vi "Iterator.vi"(8 "error in":errorcluster, 11 "Iterator Actor in":refnum<class "Iterator NR Actor.lvclass">) -> (0 "error out":errorcluster, 3 "Iterator Actor out":refnum<class "Iterator NR Actor.lvclass">)   [LabVIEW 2023, in "Iterator Actor.lvlib" / "Iterator NR Actor.lvclass"]
doc: "(<B>Filename</B>: Actor Framework.lvlib:Actor.lvclass:Actor Core.vi)\n\nReceives messages to the actor, reacts to them, and initiates any error handling that may shut the actor down.\n\nDescendant classes may override this VI to append parallel tasks for the actor to complete while it handles messages. Overrides use the Call Parent Method node."
uses:
  Iterator NR Actor.lvclass
  Iterator NR Actor.lvclass/Iterator NR Actor.ctl
  Abstract Iterator Actor/Abstract Iterator Actor.lvclass
  <userlib>/_OpenG.lib/error/error.llb/openg_error.lvlib
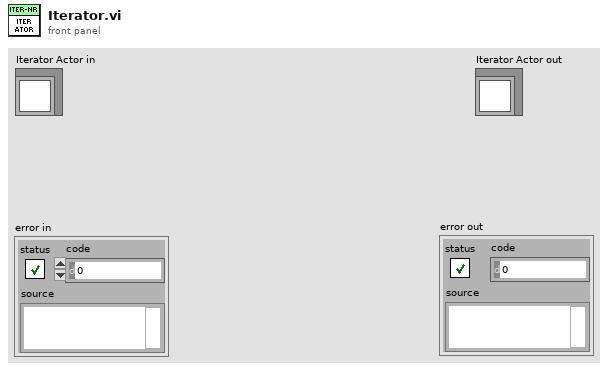
[diagram p1: front panel]
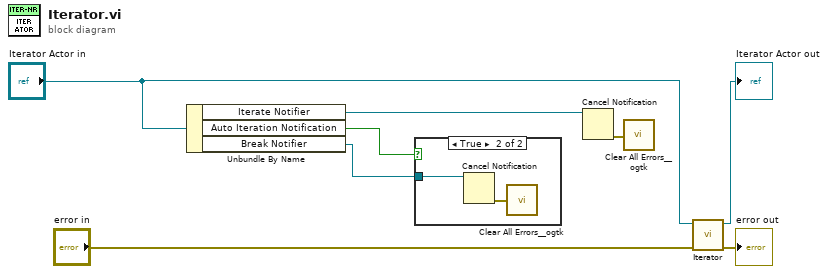
[diagram p0: block diagram]
diagram:
  n1 = Unbundle By Name("Iterator Actor in") -> ("Iterate Notifier"=w2:refnum<notifier>, "Auto Iteration Notification"=w4:bool, "Break Notifier"=w3:refnum<notifier>)
  n2 = case shown="True" w4 {
    tunnel: w3 -> [_ w10]
    frame False {
    }
    frame True {
      n3 = Cancel Notification(0:w10) -> (11:w9:errorcluster)  [unwired: 1 in, 2 out]
      n4 = call <userlib>:"Clear All Errors__ogtk.vi"("Error In"=w9) -> ()  [unwired: 3 in, 1 out]
    }
  }
  n5 = Cancel Notification(0:w2) -> (11:w1:errorcluster)  [unwired: 1 in, 2 out]
  n6 = call <userlib>:"Clear All Errors__ogtk.vi"("Error In"=w1) -> ()  [unwired: 3 in, 1 out]
  n7 = call-parent "Iterator.vi"("error in"="error in", "Iterator Actor in"="Iterator Actor in") -> ("error out"=→"error out":errorcluster, "Iterator Actor out"=→"Iterator Actor out":refnum<class "Iterator NR Actor.lvclass">)  [unwired: 8 in]
